vi "P4CMD Remove.vi"(7 "advanced options":variant, 8 "error in (no error)":errorcluster, 9 "comment":string, 10 "files":path[](array[path]), 11 "source control reference in":T1) -> (0 "error out":errorcluster, 1 "dialog box cancelled?":bool, 2 "status message":string, 3 "source control reference out":T1)   [LabVIEW 2017, in "NI_SCC_P4CMD.lvlib"]
uses:
  <vilib>/SourceControl/Providers/P4CMD/NI_SCC_P4CMD.lvlib
  <vilib>/SourceControl/sccapi/SCCAPI Refnum.ctl
  <vilib>/SourceControl/Providers/P4CMD/P4CMD Operations.ctl
  <vilib>/SourceControl/support/SCCSup Message Strings GLBL.vi
  <vilib>/SourceControl/sccapi/NI_SCC.lvlib
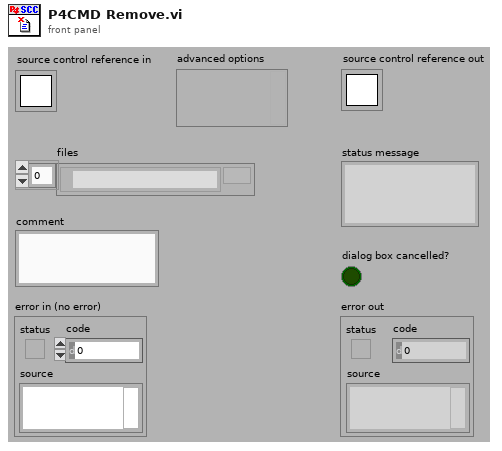
[diagram p1: front panel]
types:
  T1 = typedef "NI_SCC.lvlib/SCCAPI Refnum.ctl" = refnum<k1>
  T2 = typedef "NI_SCC_P4CMD.lvlib/P4CMD Operations.ctl" = enum16{"get all clients", "get all users", "describe changelist", "sync from depot", "open for edit", "submit to depot", "revert", "add to depot", "remove from depot", "print files revisions", "compare client file", "print depot file contents", "list opened files", "get file info", "lock files", "edit changelist spec", "info", "set variables"}
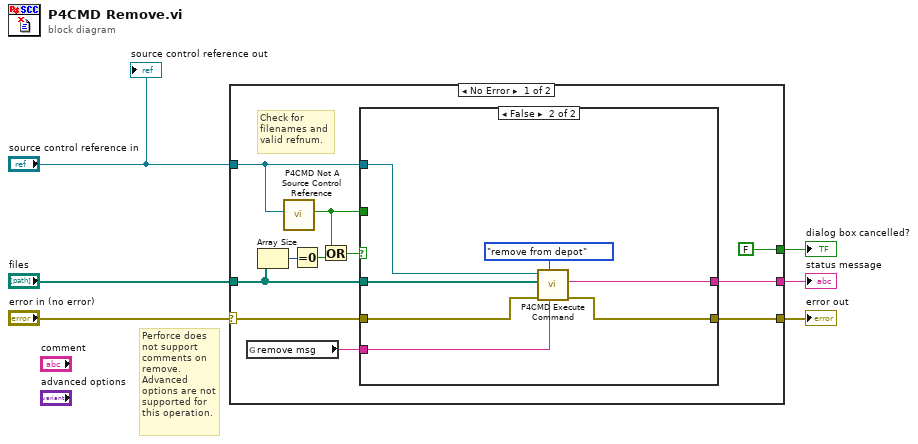
[diagram p0: block diagram]
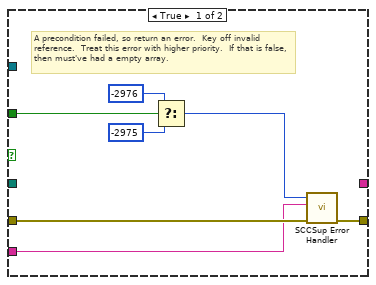
[diagram p2: hidden frame]
diagram:
  # "Perforce does not support comments on remove.  Advanced options are not supported for this operation."
  n1 = case shown="No Error" "error in (no error)" {
    selector: "error in (no error)" -> [w9 w32]
    tunnel: [w8 w32] -> w5
    tunnel: "source control reference in" -> [w14 _]
    tunnel: [w17 _] -> w3
    tunnel: "files" -> [w13 _]
    tunnel: [FALSE _] -> w1
    frame No Error {
      # "Check for filenames and valid refnum."
      n2 = global read "SCCSup Message Strings GLBL.vi" "remove msg"() -> (w7:string)
      n3 = Array Size(array=w13) -> (size(s)=w16:i32)
      n4 = call <vilib>:"P4CMD Not A Source Control Reference.vi"("source control reference in"=w14) -> ("not a source control reference?"=w11:bool)  [unwired: 9 in, 1 out]
      n5 = Equal To 0?(x=w16) -> (x = 0?=w15:bool)
      n6 = Or(x=w11, y=w15) -> (x .or. y?=w12:bool)
      n7 = case shown="False" w12 {
        tunnel: w14 -> [_ w30]
        tunnel: [_ w26] -> w17
        tunnel: w13 -> [_ w29]
        tunnel: w11 -> [w22 _]
        tunnel: w9 -> [w19 w28]
        tunnel: [w21 w27] -> w8
        tunnel: w7 -> [w18 w25]
        frame True {
          # "A precondition failed, so return an error.  Key off invalid reference.  Treat this error with higher priority.  If that is false, then must've had a empty array."
          n8 = Select(t=-2976 ("result"), s=w22, f=-2975 ("result")) -> (s? t:f=w20:i32)
          n9 = call <vilib>:"SCCSup Error Handler.vi"("error in (no error)"=w19, "operation message"=w18, "scc error code"=w20) -> ("error out"=w21:errorcluster)  [unwired: 8 in]
        }
        frame False {
          n10 = call <vilib>:"P4CMD Execute Command.vi"("operation message"=w25, "p4 operation"=P4CMD_Operations."remove from depot", "error in (no error)"=w28, "files"=w29, "source control reference in"=w30) -> ("error out"=w27:errorcluster, "command information"=w26:string)  [unwired: 4 in, 1 out]
        }
      }
    }
    frame Error {
    }
  }
  "error out" <- w5
  "status message" <- w3
  "dialog box cancelled?" <- w1
  "source control reference out" <- "source control reference in"
